vi "Extract_by_name.vi"(10 "Rsync dump":string="2015/10/28 14:16:49 [19596] receiving file list\n2015/10/28 14:18:13 [23836] .d..t...... ./\n2015/10/28 14:18:13 [23836] cd+++++++++ 20151028/\n2015/10/28 14:18:13 [23836] cd+++++++++ 20151028/20151028-181602189_dev0/\n2015/10/28 14:18:13 [23836] >f+++++++++ 20151028/20151028-181602189_dev0/20151028-181602189-000_dev0.fits\n2015/10/28 14:18:13 [23836] >f+++++++++ 20151028/20151028-181602189_dev0/20151028-181603749-001_dev0.fits\n2015/10/28 14:18:13 [23836] sent 260 bytes  received 16819795 bytes  160957.46 bytes/sec\n2015/10/28 14:18:13 [23836] total size is 4944772800  speedup is 293.98\n", 11 "Path to append to":path=path "C:/DATA/LABVIEW_TESTING") -> (1 "fULL PATH fits FILES":path[](array[path]), 2 "filenames":string[](array[string]), 3 "appended path":path)   [LabVIEW 2012]
panel:
  out "Array 2":string[](array[string])
  out "Array":i32[](array[numeric])
  out "Substrings":string[](array[string])
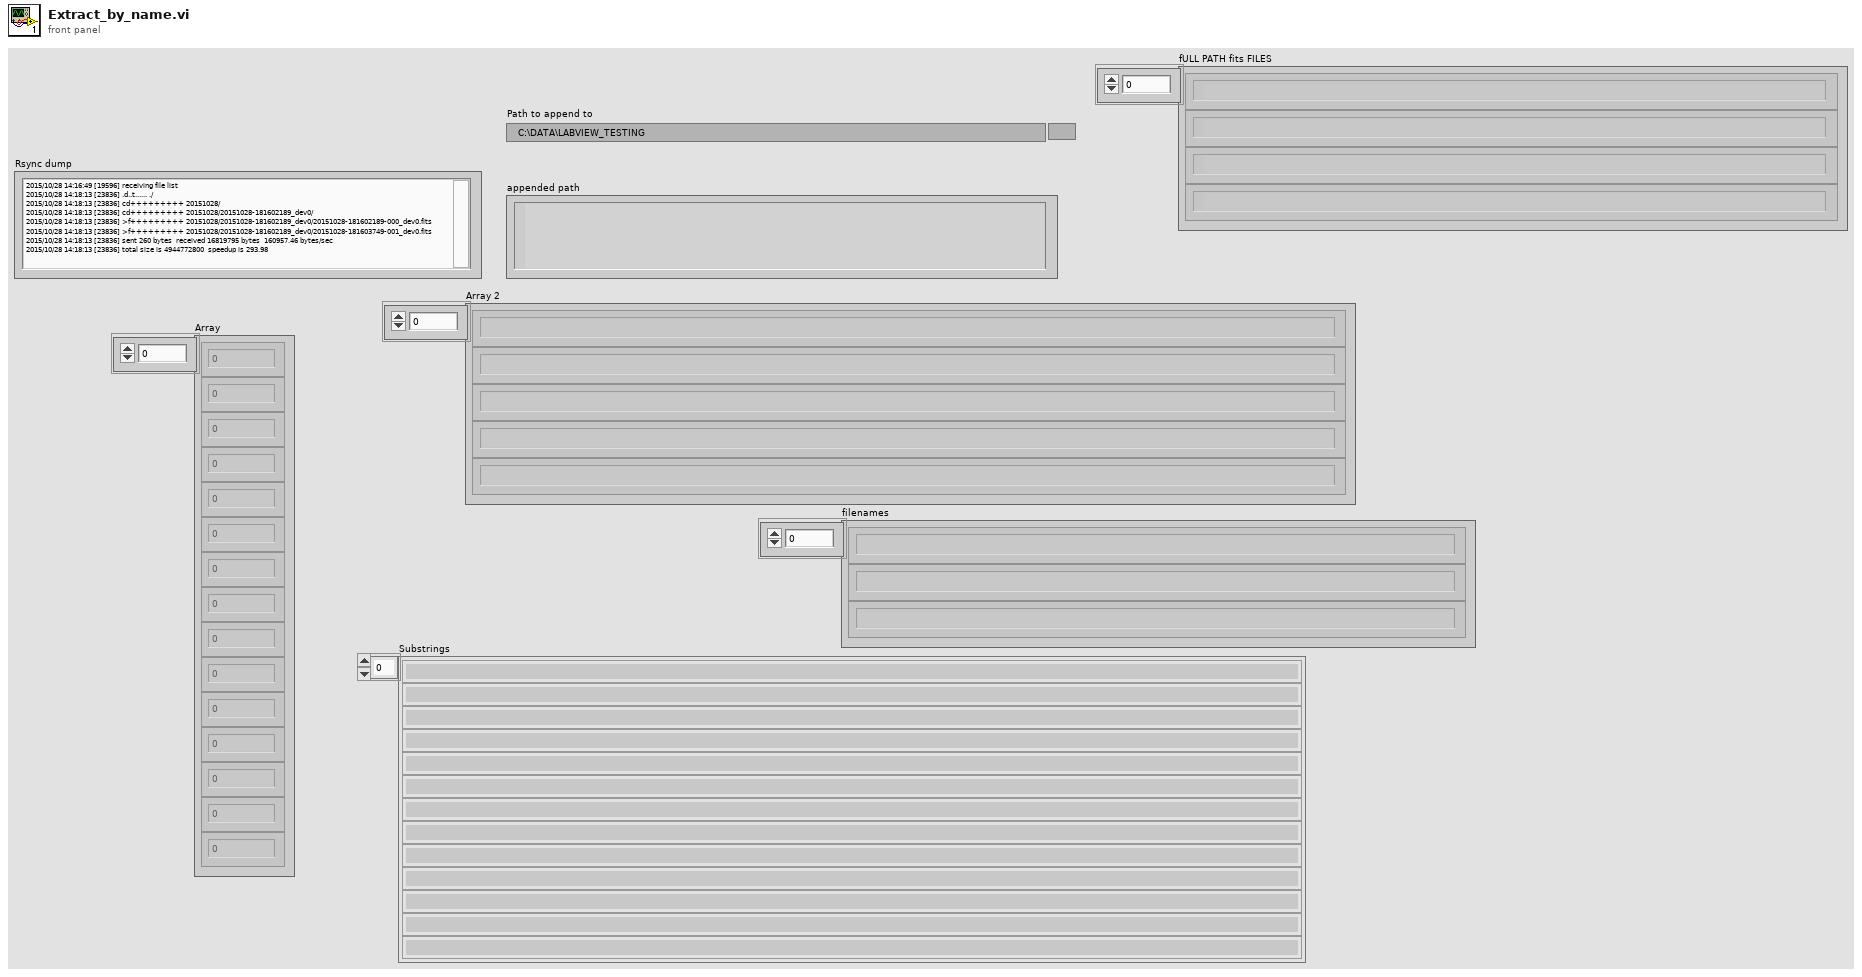
[diagram p1: front panel]
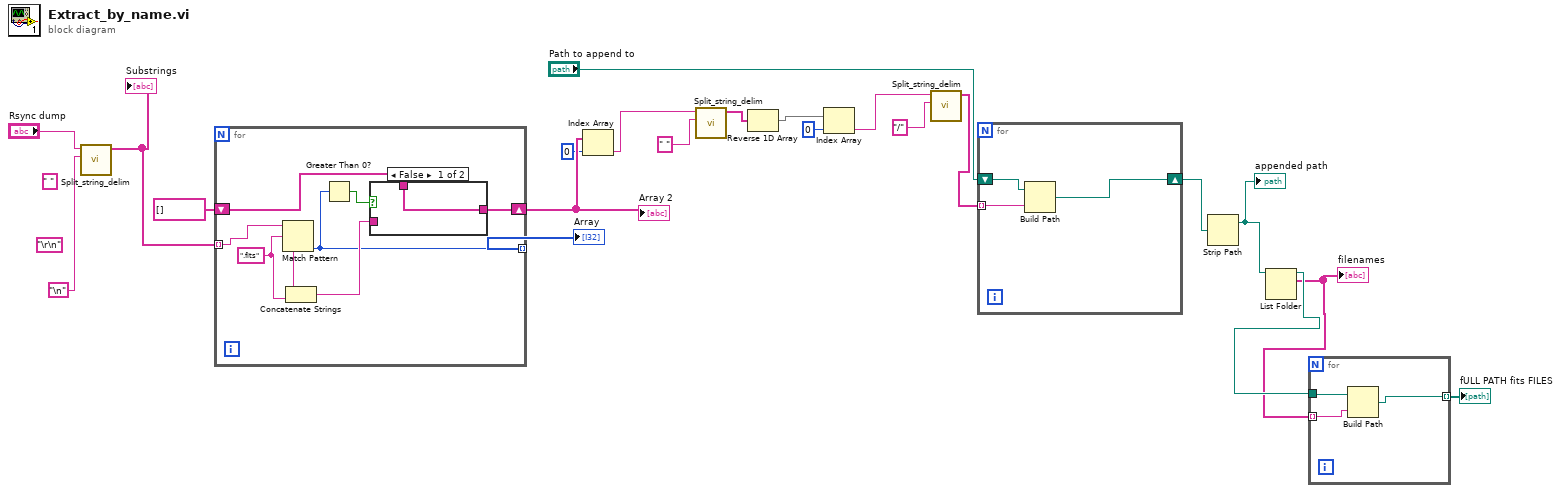
[diagram p0: block diagram]
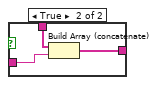
[diagram p2: hidden frame]
diagram:
  (unwired) "\r\n"
  (unwired) " " ("delimiter (Tab)")
  n1 = call "Split_string_delim.vi"("Delimiter"="\n", "Input String"="Rsync dump") -> ("Substrings"=w19:string[])  [unwired: 5 in, 4 out]
  "Substrings" <- w19
  n2 = for {
    tunnel: w19 -> [w29] mode=indexing
    tunnel: [w25] -> w18 mode=indexing
    shift-right: [w23] -> w16
    shift-left: string[] [] -> [w22]
    w27 = ".fits" ("regular expression")
    n3 = Match Pattern(string=w29, regular expression=w27) -> (before substring=w28:string, offset past match=w25:i32)  [unwired: 1 in, 2 out]
    n4 = Concatenate Strings(w28, w27) -> (w26:string)
    n5 = Greater Than 0?(x=w25) -> (x > 0?=w24:bool)
    n6 = case shown="False" w24 {
      tunnel: w26 -> [_ w33]
      tunnel: [w30 w32] -> w23
      tunnel: w22 -> [w30 w31]
      frame False {
      }
      frame True {
        n7 = Build Array (concatenate)(w31, w33) -> (w32:string[])
      }
    }
  }
  "Array" <- w18
  "Array 2" <- w16
  n8 = Index Array(array=w16, index=0) -> (element=w14:string)
  n9 = call "Split_string_delim.vi"("Delimiter"=" " ("delimiter (Tab)"), "Input String"=w14) -> ("Substrings"=w12:string[])  [unwired: 5 in, 4 out]
  n10 = Reverse 1D Array(array=w12) -> (reversed array=w10:string[])
  n11 = Index Array(array=w10, index=0) -> (element=w8:string)
  n12 = call "Split_string_delim.vi"("Delimiter"="/" ("delimiter (Tab)"), "Input String"=w8) -> ("Substrings"=w6:string[])  [unwired: 5 in, 4 out]
  n13 = for {
    tunnel: w6 -> [w34] mode=indexing
    shift-right: [w35] -> w5
    shift-left: "Path to append to" -> [w36]
    n14 = Build Path(base path=w36, name or relative path=w34) -> (appended path=w35:path)
  }
  n15 = Strip Path(path=w5) -> (stripped path=w4:path)  [unwired: 1 out]
  "appended path" <- w4
  n16 = List Folder(path=w4) -> (path out=w3:path, filenames=w2:string[])  [unwired: 3 in, 2 out]
  "filenames" <- w2
  n17 = for {
    tunnel: w3 -> [w39]
    tunnel: w2 -> [w38] mode=indexing
    tunnel: [w37] -> w1 mode=indexing
    n18 = Build Path(base path=w39, name or relative path=w38) -> (appended path=w37:path)
  }
  "fULL PATH fits FILES" <- w1
